vi "FGV Timer.vi"(8 "Error In":errorcluster, 9 "Timer Mode":T1, 10 "Time Target (s)":dbl) -> (0 "Error Out":errorcluster, 1 "Time has Elapsed?":bool, 2 "Elapsed Time":dbl)   [LabVIEW 2018]
doc: "This FGV is used to control time operations. It could be used to pause an operation if some condition is met."
uses:
  Controls/FGV Timer Control.ctl
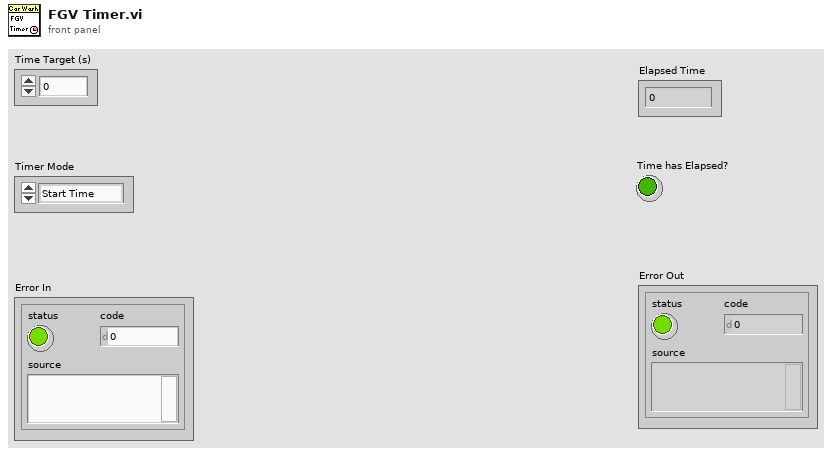
[diagram p1: front panel]
types:
  T1 = typedef "FGV Timer Control.ctl" = enum16{"Start Time", "Read Time", "Pause", "Resume"}
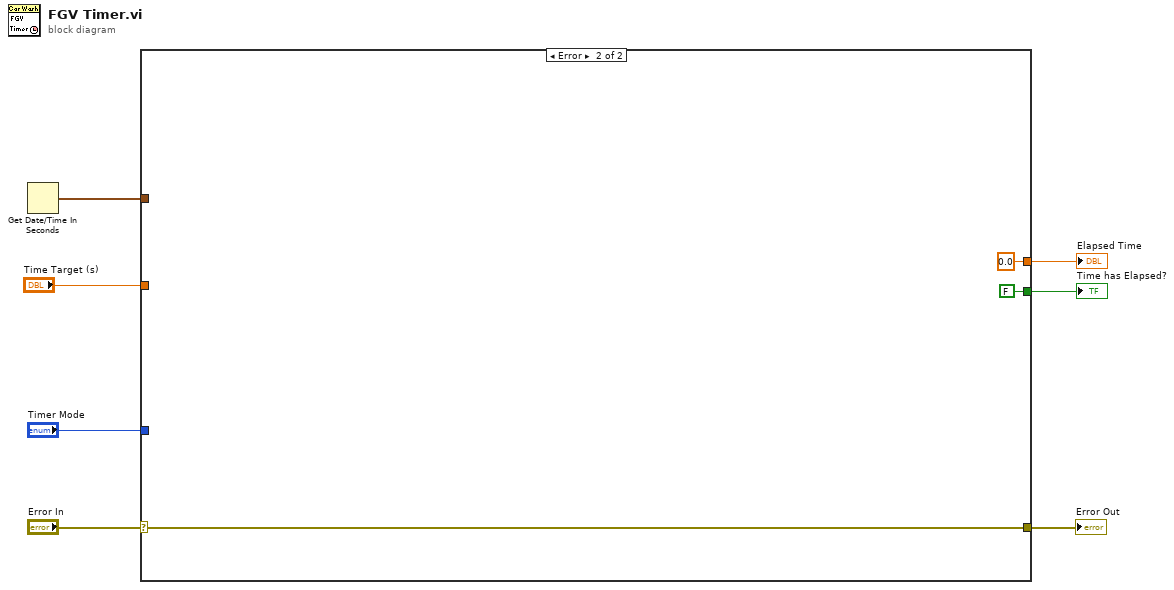
[diagram p0: block diagram]
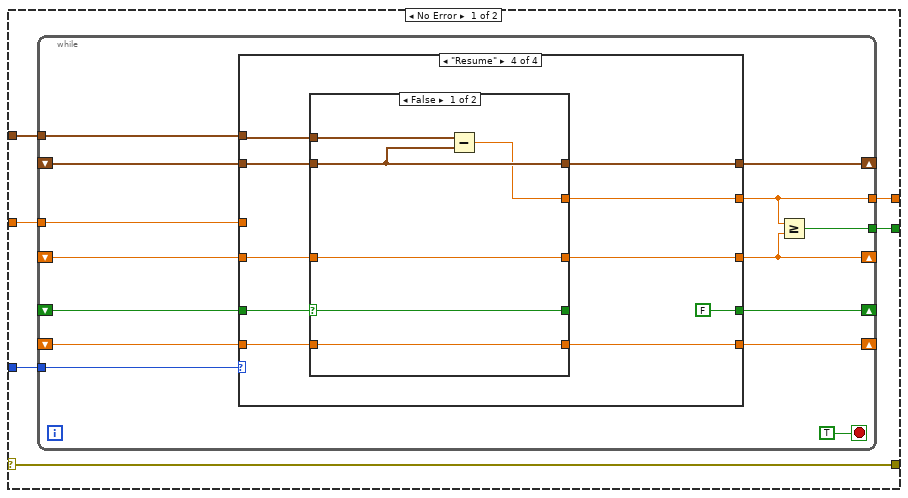
[diagram p2: hidden frame]
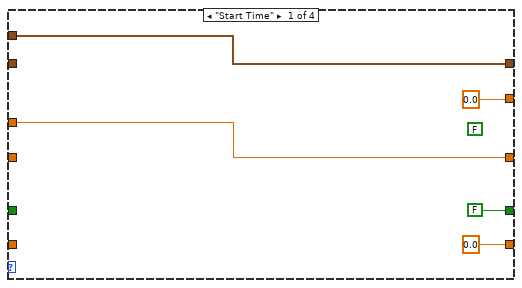
[diagram p3: hidden frame]
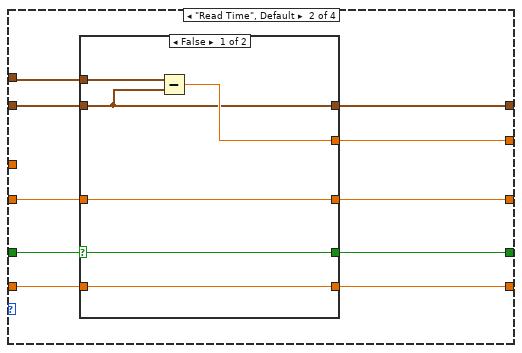
[diagram p4: hidden frame]
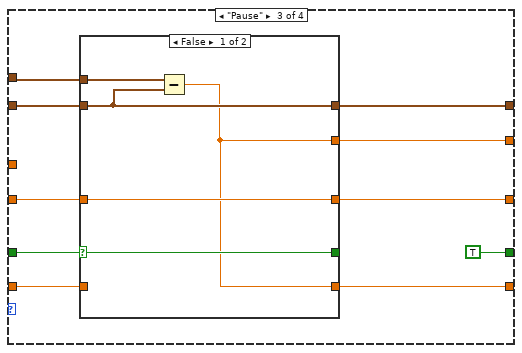
[diagram p6: hidden frame]
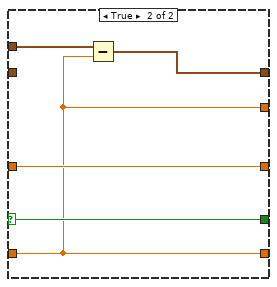
[diagram p8: hidden frame]
diagram:
  n1 = Get Date/Time In Seconds() -> (seconds since 1Jan1904=w4:timestamp)
  n2 = case shown="Error" "Error In" {
    selector: "Error In" -> [w13 w95]
    tunnel: [w13 w95] -> w6
    tunnel: "Timer Mode" -> [w12 _]
    tunnel: w4 -> [w11 _]
    tunnel: "Time Target (s)" -> [w10 _]
    tunnel: [w9 0.0] -> w2
    tunnel: [w8 FALSE] -> w1
    frame No Error {
      n3 = while {
        tunnel: w12 -> [w26]
        tunnel: w11 -> [w25]
        shift-right: [w24] -> _
        shift-left: _ -> [w23]
        tunnel: w10 -> [w22]
        shift-right: [w14] -> _
        shift-left: _ -> [w21]
        tunnel: [w15] -> w9
        tunnel: [w16] -> w8
        shift-right: [w20] -> _
        shift-left: _ -> [w18]
        shift-right: [w19] -> _
        shift-left: _ -> [w17]
        stop <- TRUE stop-if-true
        n4 = case shown="\"Resume\"" w26 {
          tunnel: w25 -> [w32 w42 w62 w81]
          tunnel: [w32 w39 w59 w78] -> w24
          tunnel: w23 -> [_ w41 w61 w80]
          tunnel: w22 -> [w31 _ _ _]
          tunnel: [w31 w37 w57 w76] -> w14
          tunnel: w21 -> [_ w38 w58 w77]
          tunnel: [0.0 w40 w60 w79] -> w15
          tunnel: [FALSE w35 TRUE FALSE] -> w20
          tunnel: [0.0 w34 w55 w74] -> w19
          tunnel: w18 -> [_ w36 w56 w75]
          tunnel: w17 -> [_ w33 w54 w73]
          frame "Start Time" {
            (unwired) FALSE
          }
          frame "Read Time", Default {
            n5 = case shown="False" w36 {
              selector: w36 -> [w44 w49]
              tunnel: w42 -> [w48 _]
              tunnel: w41 -> [w46 w52]
              tunnel: [w47 w51] -> w40
              tunnel: [w46 w52] -> w39
              tunnel: w38 -> [w45 w50]
              tunnel: [w45 w50] -> w37
              tunnel: [w44 w49] -> w35
              tunnel: [w43 w51] -> w34
              tunnel: w33 -> [w43 w51]
              frame False {
                n6 = Subtract(x=w48, y=w46) -> (x-y=w47:dbl)
              }
              frame True {
              }
            }
          }
          frame "Pause" {
            n7 = case shown="False" w56 {
              selector: w56 -> [w64 w68]
              tunnel: w62 -> [w67 _]
              tunnel: w61 -> [w66 w71]
              tunnel: [w63 w70] -> w60
              tunnel: [w66 w71] -> w59
              tunnel: w58 -> [w65 w69]
              tunnel: [w65 w69] -> w57
              tunnel: [w64 w68] -> _
              tunnel: [w63 w70] -> w55
              tunnel: w54 -> [_ w70]
              frame False {
                n8 = Subtract(x=w67, y=w66) -> (x-y=w63:dbl)
              }
              frame True {
              }
            }
          }
          frame "Resume" {
            n9 = case shown="False" w75 {
              selector: w75 -> [w85 w90]
              tunnel: w81 -> [w84 w92]
              tunnel: w80 -> [w83 _]
              tunnel: [w82 w89] -> w79
              tunnel: [w83 w88] -> w78
              tunnel: w77 -> [w86 w91]
              tunnel: [w86 w91] -> w76
              tunnel: [w85 w90] -> _
              tunnel: [w87 w89] -> w74
              tunnel: w73 -> [w87 w89]
              frame False {
                n10 = Subtract(x=w84, y=w83) -> (x-y=w82:dbl)
              }
              frame True {
                n11 = Subtract(x=w92, y=w89) -> (x-y=w88:timestamp)
              }
            }
          }
        }
        n12 = Greater Or Equal?(x=w15, y=w14) -> (x >= y?=w16:bool)
      }
    }
    frame Error {
    }
  }
  "Error Out" <- w6
  "Elapsed Time" <- w2
  "Time has Elapsed?" <- w1
